vi "Robot Global Data.vi"() -> ()   [LabVIEW 2017]
doc: "This global VI can contain as many global variables as you need. To create a global variable, place a control on the panel, give it a good name. To read or write to it from a VI, drag the icon to the diagram of that VI. You can also drag from the project. Click on the node to change which global you access. You shouldn't have multiple locations writing to a global or it will cause a race-condition."
uses:
  <vilib>/Rock Robotics/WPI/Camera/WPI_CameraImageSize.ctl
  <vilib>/Rock Robotics/WPI/DriverStation/WPI_DriverStationRobotMode2.ctl
  Support Code/Gyro/Gyro_TypeDef.ctl
  Support Code/Joysticks/Generic/Joystick_Generic_0_Data.ctl
  Support Code/Joysticks/XBox/Joystick_XBox_0_Data.ctl
  Support Code/DriverStation_TypeDef.ctl
  <vilib>/Rock Robotics/WPI/DriverStation/WPI_DriverStationAllianceInfo.ctl
  <vilib>/Rock Robotics/WPI/DriverStation/WPI_DriverStationPositionInfo.ctl
panel:
  in  "Gyro_Zero":bool
  out "Gyro_Data":T1
  out "DriverStation_Data":T2
  out "Joystick_XBox_0_Data":T5
  out "Joystick_Generic_0_Data":T6
  in  "image size":T7=enum."320x240"
  in  "Enable Vision":bool
  in  "Robot Mode":T8
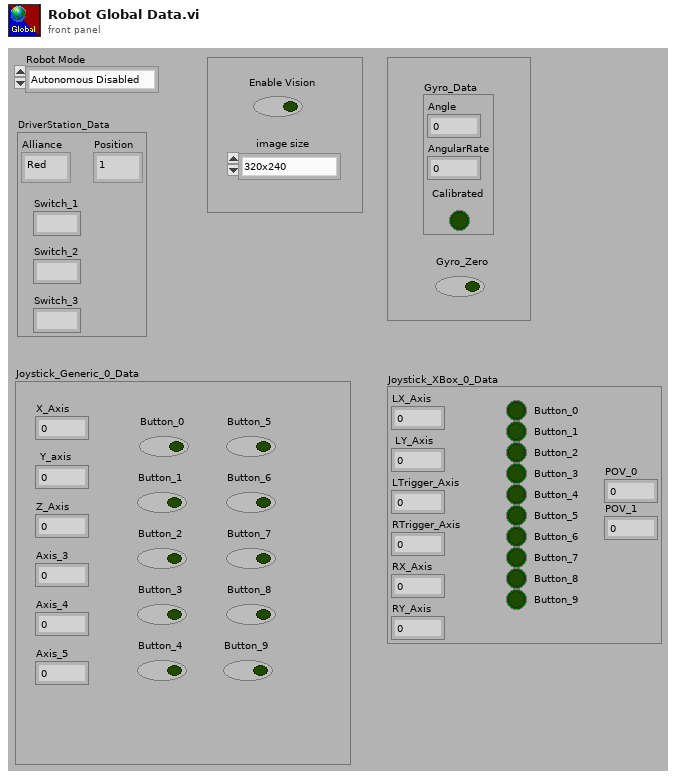
[diagram p1: front panel]
types:
  T1 = typedef "Gyro_TypeDef.ctl" = cluster{"Angle":dbl, "AngularRate":dbl, "Calibrated":bool}
  T2 = typedef "DriverStation_TypeDef.ctl" = cluster{"Alliance":T3, "Position":T4, "Switch_1":string, "Switch_2":string, "Switch_3":string}
  T3 = typedef "WPI_DriverStationAllianceInfo.ctl" = enum16{"Red", "Blue", "Invalid"}
  T4 = typedef "WPI_DriverStationPositionInfo.ctl" = enum16{"1", "2", "3"}
  T5 = typedef "Joystick_XBox_0_Data.ctl" = cluster{"LX_Axis":dbl, "LY_Axis":dbl, "LTrigger_Axis":dbl, "RTrigger_Axis":dbl, "RX_Axis":dbl, "RY_Axis":dbl, "Button_0":bool, "Button_1":bool, "Button_2":bool, "Button_3":bool, "Button_4":bool, "Button_5":bool, "Button_6":bool, "Button_7":bool, "Button_8":bool, "Button_9":bool, "POV_0":i16, "POV_1":i16}
  T6 = typedef "Joystick_Generic_0_Data.ctl" = cluster{"X_Axis":dbl, "Y_axis":dbl, "Z_Axis":dbl, "Axis_3":dbl, "Axis_4":dbl, "Axis_5":dbl, "Button_0":bool, "Button_1":bool, "Button_2":bool, "Button_3":bool, "Button_4":bool, "Button_5":bool, "Button_6":bool, "Button_7":bool, "Button_8":bool, "Button_9":bool}
  T7 = typedef "WPI_CameraImageSize.ctl" = enum16{"640x480", "320x240", "160x120", "Custom"}
  T8 = typedef "WPI_DriverStationRobotMode2.ctl" = enum16{"Autonomous Disabled", "Autonomous Enabled", "Teleop Disabled", "Teleop Enabled", "Disconnected", "Finish", "Test Disabled", "Test Enabled", "Emergency Stopped"}
diagram:
